vi "Find Wire To-From.vi"(9 "Wires":T1[](array[typedef]), 10 "termUUID":string, 11 "From UUID?":bool) -> (2 "Index":i32, 3 "Wire":T1)   [LabVIEW 2025]
uses:
  wire.ctl
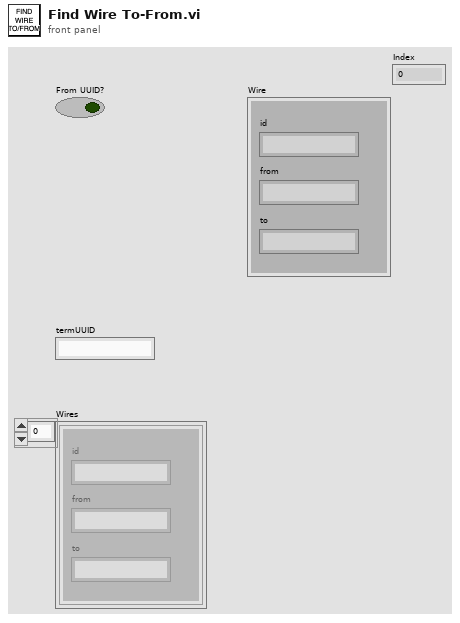
[diagram p1: front panel]
types:
  T1 = typedef "wire.ctl" = cluster{"id":string, "from":string, "to":string}
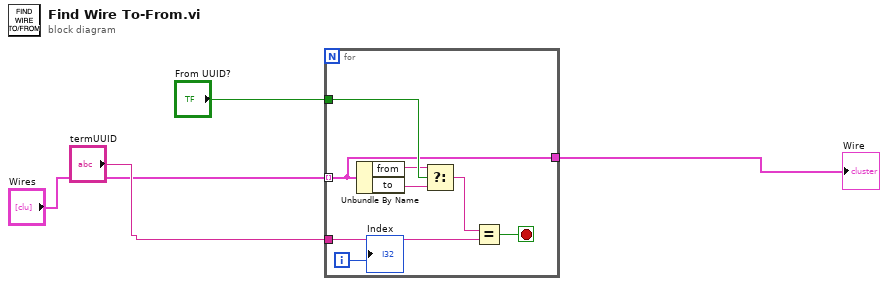
[diagram p0: block diagram]
diagram:
  n1 = for {
    tunnel: "Wires" -> [w7] mode=indexing
    tunnel: "From UUID?" -> [w12]
    tunnel: "termUUID" -> [w8]
    tunnel: [w7] -> w4
    i -> [w5]
    stop <- w6 stop-if-true
    n2 = Unbundle By Name(w7) -> ("from"=w10:string, "to"=w11:string)
    n3 = Select(t=w10, s=w12, f=w11) -> (s? t:f=w9:string)
    n4 = Equal?(x=w9, y=w8) -> (x = y?=w6:bool)
    "Index" <- w5
  }
  "Wire" <- w4
